vi "Set Parameter.vi"(8 "error in (no error)":errorcluster, 9 "Value":string, 10 "Property":string, 11 "TDCManager":T1) -> (0 "error out":errorcluster, 3 "TDCManager":T1)   [LabVIEW 2016, in "HPTDC Driver Library.lvlib"]
uses:
  HPTDC Driver Library.lvlib
  Typedefs/TDCManager.ctl
  C:/Users/CRT Controller/CRTC Labview Application/Source/HPTDC Driver Library Folder/Library files/hptdc_net4_3.7.0_x64.dll
  hptdc_net4_3.7.0_x64.dll
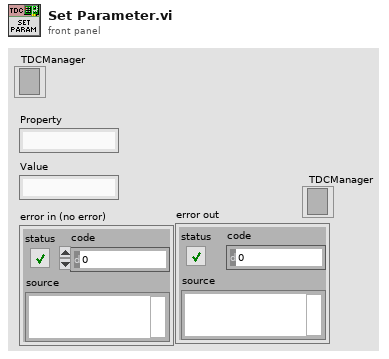
[diagram p1: front panel]
types:
  T1 = typedef "HPTDC Driver Library.lvlib/TDCManager.ctl" = refnum<k24>
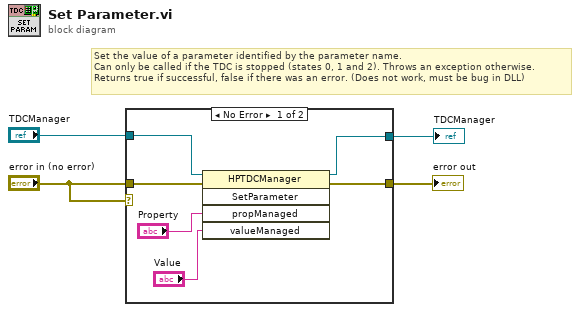
[diagram p0: block diagram]
diagram:
  # "Set the value of a parameter identified by the parameter name.\nCan only be called if the TDC is stopped (states 0, 1 and 2). Throws an exception otherwise.\nReturns true if successful, false if there was an error. (Does not work, must be bug in DLL)"
  n1 = case shown="No Error" "error in (no error)" {
    tunnel: "error in (no error)" -> [w10 w12]
    tunnel: [w9 w12] -> w4
    tunnel: [w8 w11] -> w3
    tunnel: "TDCManager" -> [w7 w11]
    frame No Error {
      n2 = invoke class="HPTDCManager" method="SetParameter"(reference=w7, error in=w10, "propManaged"="Property", "valueManaged"="Value") -> (reference out=w8:T1, error out=w9:errorcluster)  [unwired: 1 in, 3 out]
    }
    frame Error {
    }
  }
  "error out" <- w4
  "TDCManager" <- w3
